vi "Continuous ERD Write.vi"(0 "GEA2 Reference In":refnum<k24>, 1 "GEA Inputs":T1={"Source"=228, "Destination"=0} {"Destination" format="%.0x"; "Source" format="%.0x"}, 5 "Queue Name":string="ERD Write 1", 7 "Rate (s)":i32=250, 9 "Write ERD List":T2[](array[typedef]) {"ERD Number" format="%.0x"}, 11 "Error In":errorcluster, 12 "Verify ERD Response?":bool=TRUE) -> (4 "GEA2 Reference Out":refnum<k24>, 15 "Error Out":errorcluster)   [LabVIEW 2016]
doc: "This VI continuously writes an array of ERDs at a specified rate. The VI is reentrant and can be called asynchronously from TestStand. Multiple copies of the VI can be started and controlled by giving each a different Queue name. If the same name is given then multiples copies can be run, but will be stopped at the same time when stop is called."
uses:
  LabVIEW_GEA2_Toolkit.lvlibp/type defs/ERD Write Data In.ctl
  LabVIEW_GEA2_Toolkit.lvlibp/type defs/Data Type.ctl
  Q:/Common/DLLs/GEA3/GeaCommunication.dll
  DLLs/GEA3/GeaCommunication.dll
  LabVIEW_GEA2_Toolkit.lvlibp/type defs/Source_Destination.ctl
  LabVIEW_GEA2_Toolkit.lvlibp
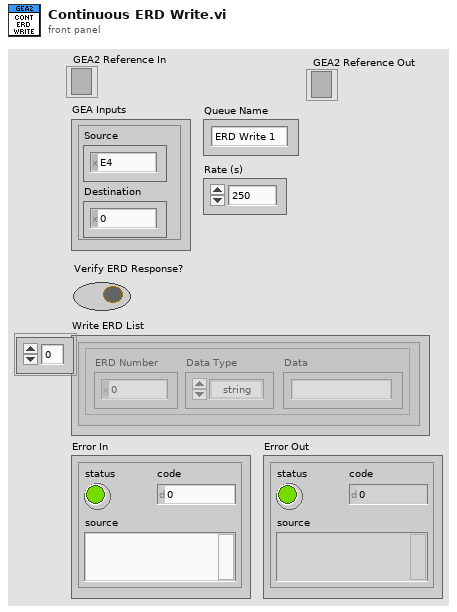
[diagram p1: front panel]
types:
  T1 = typedef "LabVIEW_GEA2_Toolkit.lvlibp/Source_Destination.ctl" = cluster{"Source":u8, "Destination":u8}
  T2 = typedef "LabVIEW_GEA2_Toolkit.lvlibp/ERD Write Data In.ctl" = cluster{"ERD Number":u16, "Data Type":T3, "Data":string}
  T3 = typedef "LabVIEW_GEA2_Toolkit.lvlibp/Data Type.ctl" = enum16{"string", "boolean", "uint8_t", "uint16_t", "uint32_t", "uint64_t", "int8_t", "int16_t", "int32_t", "int64_t"}
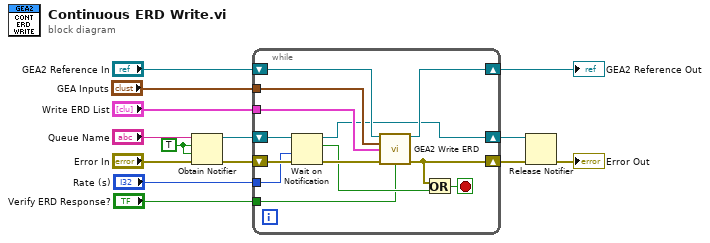
[diagram p0: block diagram]
diagram:
  w10 = TRUE ("create if not found? (T)")
  n1 = Obtain Notifier(name (unnamed)="Queue Name", notification data type=w10, create if not found? (T)=w10, error in (no error)="Error In") -> (notifier out=w14:refnum<notifier>, error out=w13:errorcluster)  [unwired: 1 out]
  n2 = while {
    tunnel: "Write ERD List" -> [w25]
    shift-right: [w18] -> w5
    shift-left: w13 -> [w26]
    tunnel: "Rate (s)" -> [w20]
    shift-right: [w19] -> w2
    shift-left: "GEA2 Reference In" -> [w21]
    tunnel: "GEA Inputs" -> [w17]
    shift-right: [w16] -> w3
    shift-left: w14 -> [w27]
    tunnel: "Verify ERD Response?" -> [w15]
    stop <- w22 stop-if-true
    n3 = Wait on Notification(notifier=w27, timeout in ms (-1)=w20, error in (no error)=w26) -> (notifier out=w16:refnum<notifier>, notification=w23:bool, error out=w24:errorcluster)  [unwired: 1 in, 1 out]
    n4 = call "GEA2 Write ERD.vi"("GEA2 Reference In"=w21, "GEA Inputs"=w17, "Write ERD List"=w25, "Error In"=w24, "Verify ERD Response?"=w15) -> ("GEA2 Reference Out"=w19:refnum<k24>, "Error Out"=w18:errorcluster)  [unwired: 8 in, 1 out]
    n5 = Or(x=w18, y=w23) -> (x .or. y?=w22:bool)
  }
  "GEA2 Reference Out" <- w2
  n6 = Release Notifier(notifier=w3, error in (no error)=w5) -> (error out=→"Error Out":errorcluster)  [unwired: 1 in, 2 out]
